vi "3ToteAuton.vi"   [LabVIEW 2014]
uses:
  TeleopCmd.ctl
  CmdFlag.ctl
types:
  T1 = typedef "TeleopCmd.ctl" = cluster{"CmdFlag":T2, "throttle":dbl, "turn":dbl, "Override":bool, "Strafe":dbl, "MotorPwrMax":u8, "Time":u32}
  T2 = typedef "CmdFlag.ctl" = enum16{"noop", "logflag", "suspend", "resume"}
  T3 = typedef "WPI_MotorControlDeviceRef.ctl" = cluster{"DeviceStatus":errorcluster, "Type":T4, "PWM":cluster{"Controller":T5, "PWM Channel":T6, "DeadBand":T7}, "CAN":cluster{"Device Number":u8, "Control Mode":T8, "Semaphore":T9, "Max Vout":dbl, "TalonSRX Control Mode":T10}, "Invert":bool, "TransformRef":T11, "InvTransformRef":T11}
  T4 = typedef "WPI_MotorControlType.ctl" = enum16{"PWM", "CAN", "CANTalonSRX"}
  T5 = typedef "FPGA_TypedefDigitalModule.ctl" = enum16{"Controller 1"}
  T6 = typedef "FPGA_DIOPWMChannel.ctl" = enum8{"PWM 0", "PWM 1", "PWM 2", "PWM 3", "PWM 4", "PWM 5", "PWM 6", "PWM 7", "PWM 8", "PWM 9", "PWM MXP 0", "PWM MXP 1", "PWM MXP 2", "PWM MXP 3", "PWM MXP 4", "PWM MXP 5", "PWM MXP 6", "PWM MXP 7", "PWM MXP 8", "PWM MXP 9", "Invalid"}
  T7 = typedef "WPI_PWMDeadband.ctl" = cluster{"Name":string, "maxPositivePwm":i32, "minPositivePwm":i32, "centerPwm":i32, "maxNegativePwm":i32, "minNegativePwm":i32, "angularRange":u16}
  T8 = typedef "WPI_CANJaguar_ControlMode.ctl" = enum8{"Percent VBus", "Current", "Speed", "Position", "Voltage"}
  T9 = typedef "Semaphore RefNum" = refnum<k1>
  T10 = typedef "WPI_CANTalonSRX_APIControlMode.ctl" = enum8{"Percent VBus", "Speed", "Position", "Slave", "Unchanged / Invalid"}
  T11 = typedef "WPI_PWMTransform_ConPane.ctl" = refnum<vi>
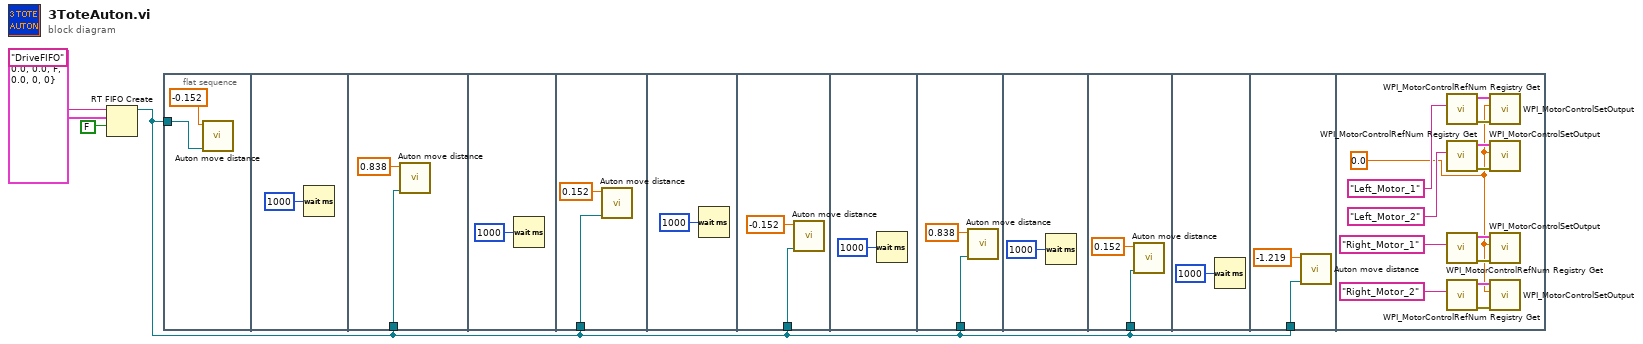
[diagram p0: block diagram]
diagram:
  n1 = RT FIFO Create(0:"DriveFIFO" ("name (unnamed)"), 1:T1 {"CmdFlag"=enum."noop", "throttle"=0.0, "turn"=0.0, "Override"=FALSE, "Strafe"=0.0, "MotorPwrMax"=0, "Time"=0} ("Cluster"), 2:FALSE ("create if not found? (T)")) -> (8:w4:refnum<k33>)  [unwired: 5 in, 2 out]
  n2 = flat-sequence {
    tunnel: w4 -> [w6]
    tunnel: w4 -> [w9]
    tunnel: w4 -> [w11]
    tunnel: w4 -> [w14]
    tunnel: w4 -> [w17]
    tunnel: w4 -> [w20]
    tunnel: w4 -> [w23]
    frame #0 {
      n3 = call "Auton move distance.vi"("Distance"=-0.152, "Refnum in"=w6) -> ()  [unwired: 8 in, 1 out]
    }
    frame #1 {
      n4 = Wait (ms)(milliseconds to wait=u32 1000) -> ()  [unwired: 1 out]
    }
    frame #2 {
      n5 = call "Auton move distance.vi"("Distance"=0.838, "Refnum in"=w9) -> ()  [unwired: 8 in, 1 out]
    }
    frame #3 {
      n6 = Wait (ms)(milliseconds to wait=u32 1000) -> ()  [unwired: 1 out]
    }
    frame #4 {
      n7 = call "Auton move distance.vi"("Distance"=0.152, "Refnum in"=w11) -> ()  [unwired: 8 in, 1 out]
    }
    frame #5 {
      n8 = Wait (ms)(milliseconds to wait=u32 1000) -> ()  [unwired: 1 out]
    }
    frame #6 {
      n9 = call "Auton move distance.vi"("Distance"=-0.152, "Refnum in"=w14) -> ()  [unwired: 8 in, 1 out]
    }
    frame #7 {
      n10 = Wait (ms)(milliseconds to wait=u32 1000) -> ()  [unwired: 1 out]
    }
    frame #8 {
      n11 = call "Auton move distance.vi"("Distance"=0.838, "Refnum in"=w17) -> ()  [unwired: 8 in, 1 out]
    }
    frame #9 {
      n12 = Wait (ms)(milliseconds to wait=u32 1000) -> ()  [unwired: 1 out]
    }
    frame #10 {
      n13 = call "Auton move distance.vi"("Distance"=0.152, "Refnum in"=w20) -> ()  [unwired: 8 in, 1 out]
    }
    frame #11 {
      n14 = Wait (ms)(milliseconds to wait=u32 1000) -> ()  [unwired: 1 out]
    }
    frame #12 {
      n15 = call "Auton move distance.vi"("Distance"=-1.219, "Refnum in"=w23) -> ()  [unwired: 8 in, 1 out]
    }
    frame #13 {
      w25 = 0.0 ("Motor Output")
      n16 = call <vilib>:"WPI_MotorControlRefNum Registry Get.vi"("refnum name"="Left_Motor_1") -> ("error out"=w36:errorcluster, "MotorControlDevRef"=w37:T3)  [unwired: 9 in]
      n17 = call <vilib>:"WPI_MotorControlRefNum Registry Get.vi"("refnum name"="Left_Motor_2") -> ("error out"=w34:errorcluster, "MotorControlDevRef"=w35:T3)  [unwired: 9 in]
      n18 = call <vilib>:"WPI_MotorControlRefNum Registry Get.vi"("refnum name"="Right_Motor_1") -> ("error out"=w32:errorcluster, "MotorControlDevRef"=w33:T3)  [unwired: 9 in]
      n19 = call <vilib>:"WPI_MotorControlRefNum Registry Get.vi"("refnum name"="Right_Motor_2") -> ("error out"=w30:errorcluster, "MotorControlDevRef"=w31:T3)  [unwired: 9 in]
      n20 = call <vilib>:"WPI_MotorControlSetOutput.vi"("error in (no error)"=w36, "Output"=w25, "MotorControlDevRef"=w37) -> ()  [unwired: 6 in, 3 out]
      n21 = call <vilib>:"WPI_MotorControlSetOutput.vi"("error in (no error)"=w34, "Output"=w25, "MotorControlDevRef"=w35) -> ()  [unwired: 6 in, 3 out]
      n22 = call <vilib>:"WPI_MotorControlSetOutput.vi"("error in (no error)"=w32, "Output"=w25, "MotorControlDevRef"=w33) -> ()  [unwired: 6 in, 3 out]
      n23 = call <vilib>:"WPI_MotorControlSetOutput.vi"("error in (no error)"=w30, "Output"=w25, "MotorControlDevRef"=w31) -> ()  [unwired: 6 in, 3 out]
    }
  }
